vi "updateState.vi"(8 "error in (no error)":errorcluster, 10 "Monochromator in":refnum<class "Monochromator.lvclass">, 11 "SettingUpState in":refnum<class "SettingUpState.lvclass">) -> (0 "error out":errorcluster, 2 "Monochromator out":refnum<class "Monochromator.lvclass">, 3 "SettingUpState out":refnum<class "SettingUpState.lvclass">)   [LabVIEW 2016, in "SettingUpState.lvclass"]
uses:
  SettingUpState.lvclass
  Monochromator/Monochromator.lvclass
  SettingUpState.lvclass/SettingUpState.ctl
  Monochromator/Monochromator.lvclass/Monochromator.ctl
  Typedefs/SWStatus.ctl
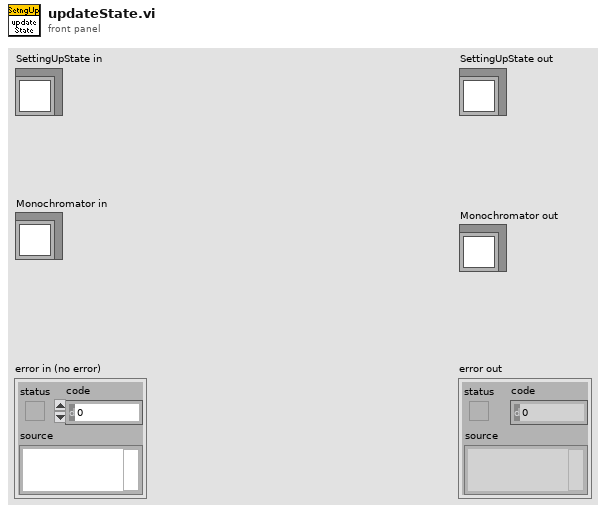
[diagram p1: front panel]
types:
  T1 = typedef "SWStatus.ctl" = enum16{"OfflineState", "ReadyState", "SettingUpState", "FaultState"}
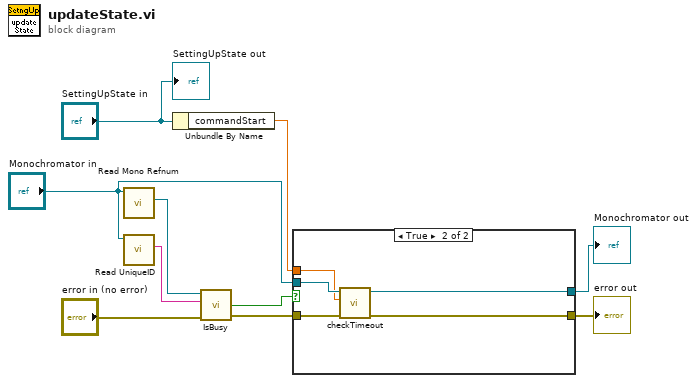
[diagram p0: block diagram]
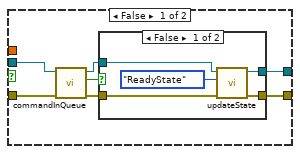
[diagram p2: hidden frame]
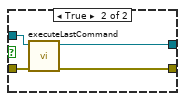
[diagram p3: hidden frame]
diagram:
  n1 = call "Read Mono Refnum.vi"("Monochromator in"="Monochromator in") -> ("Mono Refnum"=w6:refnum<k7>)  [unwired: 8 in, 2 out]
  n2 = call "Read UniqueID.vi"("Monochromator in"="Monochromator in") -> ("UniqueID"=w5:string)  [unwired: 8 in, 2 out]
  n3 = Unbundle By Name("SettingUpState in") -> ("commandStart"=w2:dbl)
  n4 = call "IsBusy.vi"("error in (no error)"="error in (no error)", "UniqueID"=w5, "RefNum In"=w6) -> ("error out"=w9:errorcluster, "IsBusy"=w1:bool)  [unwired: 1 in, 1 out]
  n5 = case shown="True" w1 {
    tunnel: [w11 w28] -> w8
    tunnel: w9 -> [w16 w29]
    tunnel: "Monochromator in" -> [w17 w31]
    tunnel: [w12 w30] -> w4
    tunnel: w2 -> [_ w27]
    frame False {
      n6 = call "commandInQueue.vi"("error in (no error)"=w16, "Monochromator in"=w17) -> ("error out"=w13:errorcluster, "commandInQueue?"=w15:bool, "Monochromator out"=w14:refnum<class "Monochromator.lvclass">)  [unwired: 7 in]
      n7 = case shown="False" w15 {
        tunnel: w14 -> [w21 w26]
        tunnel: w13 -> [w20 w25]
        tunnel: [w19 w23] -> w12
        tunnel: [w18 w24] -> w11
        frame False {
          n8 = call "updateState.vi"("error in (no error)"=w20, "SWStatus"=SWStatus."ReadyState", "Monochromator in"=w21) -> ("error out"=w18:errorcluster, "Monochromator out"=w19:refnum<class "Monochromator.lvclass">)  [unwired: 7 in]
        }
        frame True {
          n9 = call "executeLastCommand.vi"("error in (no error)"=w25, "Monochromator in"=w26) -> ("error out"=w24:errorcluster, "Monochromator out"=w23:refnum<class "Monochromator.lvclass">)  [unwired: 8 in]
        }
      }
    }
    frame True {
      n10 = call "checkTimeout.vi"("error in (no error)"=w29, "executionTime"=w27, "Monochromator in"=w31) -> ("error out"=w28:errorcluster, "Monochromator out"=w30:refnum<class "Monochromator.lvclass">)  [unwired: 6 in, 1 out]
    }
  }
  "error out" <- w8
  "Monochromator out" <- w4
  "SettingUpState out" <- "SettingUpState in"
